vi "read_As_Gas.vi"() -> (0 "H2 Flush":bool, 1 "As Gas Actual Flow Rate":dbl, 2 "Remote":bool, 3 "Run":bool, 4 "Gas In":bool, 5 "Active":bool)   [LabVIEW 2011]
uses:
  low_level_proc/globals.vi
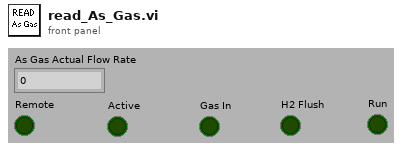
[diagram p1: front panel]
types:
  T1 = typedef "relaySpec.ctl" = cluster{"Card Index":u16, "Relay Index":u16}
  T2 = typedef "DA_Spec.ctl" = cluster{"Card Index":u16, "Channel Index":u16}
  T3 = typedef "AD_Spec.ctl" = u16
  T4 = cluster{"Relay Functions":cluster{"Remote":T1, "Active":T1, "Gas in":T1, "H2 flush":T1, "Run":T1}, "D/A Functions":cluster{"Flow":T2}, "Flow Range":cluster{"Flow (ASGMFC1)":u16}, "A/D Functions":cluster{"Flow":T3}}
  T5 = cluster{"Remote":T1, "Active":T1, "Gas in":T1, "H2 flush":T1, "Run":T1}
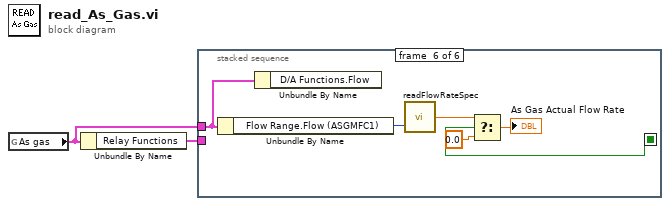
[diagram p0: block diagram]
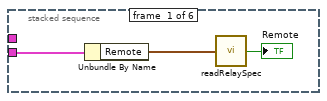
[diagram p2: hidden frame]
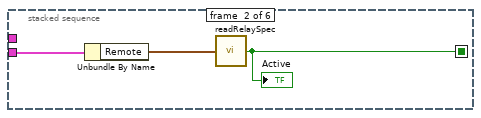
[diagram p3: hidden frame]
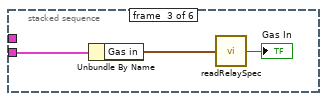
[diagram p4: hidden frame]
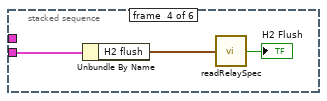
[diagram p5: hidden frame]
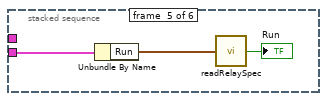
[diagram p6: hidden frame]
diagram:
  n1 = global read "globals.vi" "As gas"() -> (w1:T4)
  n2 = Unbundle By Name(w1) -> ("Relay Functions"=w2:T5)
  n3 = stacked-sequence {
    seq-local: [_ w6 _ _ _ _] -> [_ _ _ _ _ w23]
    tunnel: w2 -> [w5 w8 w10 w13 w16 _]
    tunnel: w1 -> [_ _ _ _ _ w21]
    frame #0 {
      n4 = Unbundle By Name(w5) -> ("Remote"=w4:T1)
      n5 = call "readRelaySpec.vi"("RelaySpec"=w4) -> ("Relay Status"=→"Remote":bool)
    }
    frame #1 {
      n6 = Unbundle By Name(w8) -> ("Remote"=w7:T1)
      n7 = call "readRelaySpec.vi"("RelaySpec"=w7) -> ("Relay Status"=w6:bool)
      "Active" <- w6
    }
    frame #2 {
      n8 = Unbundle By Name(w10) -> ("Gas in"=w9:T1)
      n9 = call "readRelaySpec.vi"("RelaySpec"=w9) -> ("Relay Status"=→"Gas In":bool)
    }
    frame #3 {
      n10 = Unbundle By Name(w13) -> ("H2 flush"=w14:T1)
      n11 = call "readRelaySpec.vi"("RelaySpec"=w14) -> ("Relay Status"=→"H2 Flush":bool)
    }
    frame #4 {
      n12 = Unbundle By Name(w16) -> ("Run"=w17:T1)
      n13 = call "readRelaySpec.vi"("RelaySpec"=w17) -> ("Relay Status"=→"Run":bool)
    }
    frame #5 {
      n14 = Unbundle By Name(w21) -> ("Flow Range.Flow (ASGMFC1)"=w20:u16)
      n15 = Unbundle By Name(w21) -> ()  [unwired: 1 out]
      n16 = call "readFlowRateSpec.vi"("Flow range Index"=w20) -> ("Flow Rate (sccm)"=w19:dbl)  [unwired: 1 in]
      n17 = Select(t=w19, s=w23, f=0.0) -> (s? t:f=→"As Gas Actual Flow Rate":dbl)
    }
  }
